vi "Build qREL query command substring.vi"(0 "System no.":i32=1 min=1 max=4 step=1, 2 "Relays to query in":string[](array[string]), 3 "Query\nAll relays?":bool, 4 "For all relays: use\nRelay identifier?":bool=TRUE, 5 "error in":errorcluster) -> (14 "Command substring":string, 15 "Relays to query out":string[](array[string]), 16 "Number of rows":u32=1, 19 "error out":errorcluster)   [LabVIEW 2026]
doc: "This VI builds a REL? query command substring. If Query all relays is TRUE, available relays are read using TRC?.vi and relay identifiers are assigned using TVI?.vi (valid identifiers are assigned to available relays in ascending order). Number of rows is size of the Relays to query out array. If Relay identifier is FALSE, Command substring is an empty string. \nExample: If one relay board is installed in the system to command, Relays to query in is A;B;D, Query all relays? is TRUE and Use Relay identifier is TRUE, resulting Command substring is \"ABCDEFGH\", Number of rows is 8 and Relays to query out is A;B;C;D;E;F;G;H."
panel:
  # "This vi builds a REL? query command substring. If \"Query all relays\" is true, available relays\nare read using TRC? and relay identifiers are assigned using TVI? (valid identifiers are assigned\nto available relays in ascending order). Number of rows is size of the \"Relays to query out\" array.\nIf \"Use relay identifier\" is false, command substring is an empty string."
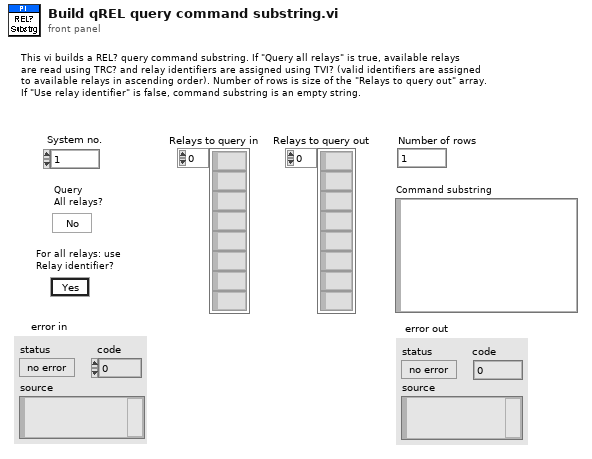
[diagram p1: front panel]
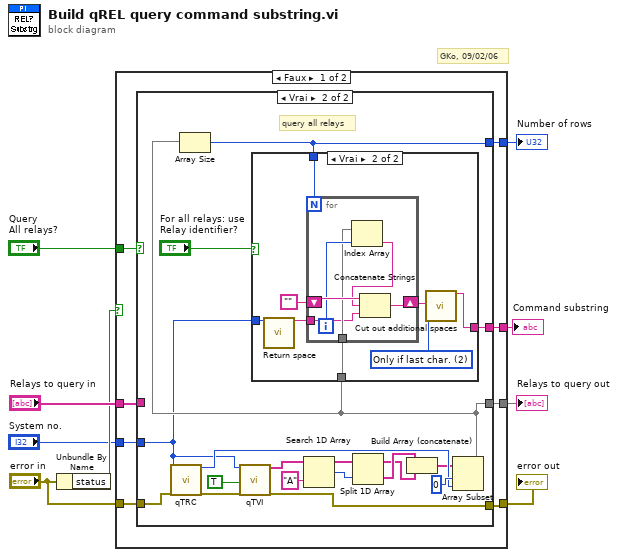
[diagram p0: block diagram]
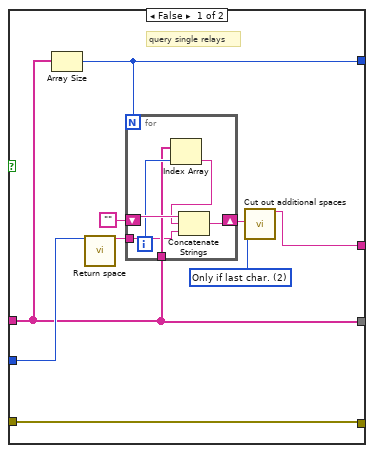
[diagram p2: hidden frame]
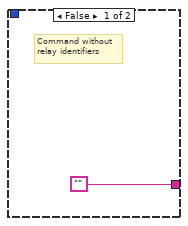
[diagram p3: hidden frame]
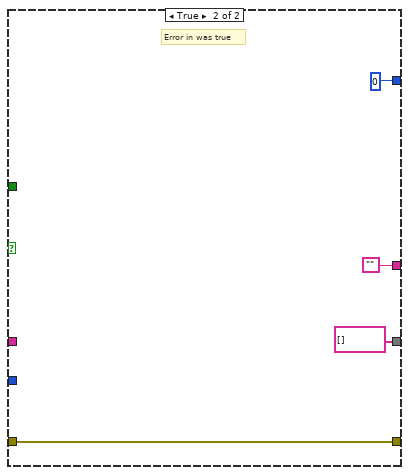
[diagram p4: hidden frame]
diagram:
  # "GKo, 09/02/06"
  n1 = Unbundle By Name("error in") -> ("status"=w4:bool)
  n2 = case shown="Faux" w4 {
    tunnel: [w17 0] -> w9
    tunnel: "Relays to query in" -> [w16 _]
    tunnel: "Query\nAll relays?" -> [w15 _]
    tunnel: [w14 string[] [] ("Relais to query in")] -> w6
    tunnel: [w13 ""] -> w5
    tunnel: [w11 w68] -> w3
    tunnel: "error in" -> [w12 w68]
    tunnel: "System no." -> [w10 _]
    frame False {
      n3 = case shown="Vrai" w15 {
        tunnel: [w18 w49] -> w13
        tunnel: w16 -> [w19 _]
        tunnel: [w19 w41] -> w14
        tunnel: [w20 w48] -> w17
        tunnel: w12 -> [w26 w46]
        tunnel: [w26 w43] -> w11
        tunnel: w10 -> [w21 w33]
        frame False {
          w23 = u16 2 items=["All Spaces", "Only if 1st char.", "Only if last char.", "Only if near \"=\"", "Only if 1st or last char.", "Only multiple"] ("Mode")
          # "query single relays"
          n4 = Array Size(array=w19) -> (size(s)=w20:i32)
          n5 = call "Return space.vi"("System no."=w21) -> ("String out"=w22:string)  [unwired: 1 in, 17 out]
          n6 = for {
            N: w20 -> [_]
            shift-right: [w31] -> w24
            shift-left: "" -> [w32]
            tunnel: w19 -> [w29]
            tunnel: w22 -> [w27]
            i -> [w30]
            n7 = Index Array(array=w29, index=w30) -> (element=w28:string)
            n8 = Concatenate Strings(w32, w28, w27) -> (w31:string)
          }
          n9 = call "Cut out additional spaces.vi"("String"=w24, "Mode"=w23) -> ("String out"=w18:string)  [unwired: 17 out]
        }
        frame True {
          # "query all relays"
          n10 = call "qTRC.vi"("System no."=w33, "error in"=w46) -> ("Number of relays"=w40:i32, "error out"=w44:errorcluster)  [unwired: 16 out]
          n11 = call "qTVI.vi"("System no."=w33, "Invert order"=TRUE, "error in"=w44) -> ("Valid axis IDs"=w35:string[], "error out"=w43:errorcluster)  [unwired: 15 out]
          n12 = Search 1D Array(1D array=w35, element="A") -> (index of element=w38:i32)  [unwired: 1 out]
          n13 = Split 1D Array(array=w35, index=w38) -> (first subarray=w36:string[], second subarray=w37:string[])
          n14 = Build Array (concatenate)(w37, w36) -> (w34:string[])
          n15 = Array Subset(array=w34, index=0 ("Array Index"), length=w40) -> (w41:string[])
          n16 = Array Size(array=w41) -> (size(s)=w48:i32)
          n17 = case shown="Vrai" "For all relays: use\nRelay identifier?" {
            tunnel: ["" w51] -> w49
            tunnel: w41 -> [_ w53]
            tunnel: w48 -> [_ w52]
            tunnel: w33 -> [_ w54]
            frame False {
              # "Command without\nrelay identifiers"
            }
            frame True {
              w56 = u16 2 items=["All Spaces", "Only if 1st char.", "Only if last char.", "Only if near \"=\"", "Only if 1st or last char.", "Only multiple"] ("Mode")
              n18 = call "Return space.vi"("System no."=w54) -> ("String out"=w55:string)  [unwired: 1 in, 17 out]
              n19 = for {
                N: w52 -> [_]
                shift-right: [w63] -> w57
                shift-left: "" -> [w64]
                tunnel: w53 -> [w61]
                tunnel: w55 -> [w59]
                i -> [w62]
                n20 = Index Array(array=w61, index=w62) -> (element=w60:string)
                n21 = Concatenate Strings(w64, w60, w59) -> (w63:string)
              }
              n22 = call "Cut out additional spaces.vi"("String"=w57, "Mode"=w56) -> ("String out"=w51:string)  [unwired: 17 out]
            }
          }
        }
      }
    }
    frame True {
      # "Error in was true"
    }
  }
  "Number of rows" <- w9
  "Relays to query out" <- w6
  "Command substring" <- w5
  "error out" <- w3
